vi "PDE Solver.vi"   [LabVIEW 2017, in "NI_PDE.lvlib"]
doc: "Solves a partial differential equation. You must manually select the polymorphic instance to use."
uses:
  <vilib>/gmath/NI_PDE.lvlib
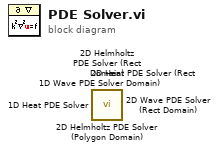
[diagram p0: block diagram]
diagram:
  n1 = call <vilib>:"2D Helmholtz PDE Solver (Polygon Domain).vi"() -> ()  [unwired: 12 in, 4 out]
  n2 = call <vilib>:"2D Heat PDE Solver (Rect Domain).vi"() -> ()  [unwired: 13 in, 3 out]
  n3 = call <vilib>:"1D Heat PDE Solver.vi"() -> ()  [unwired: 13 in, 3 out]
  n4 = call <vilib>:"2D Wave PDE Solver (Rect Domain).vi"() -> ()  [unwired: 13 in, 3 out]
  n5 = call <vilib>:"1D Wave PDE Solver.vi"() -> ()  [unwired: 13 in, 3 out]
  n6 = call <vilib>:"2D Helmholtz PDE Solver (Rect Domain).vi"() -> ()  [unwired: 13 in, 3 out]
